vi "Initialise Chmmr.vi"(8 "error in (no error)":errorcluster, 11 "Renderer":u32) -> (0 "error out":errorcluster, 2 "Deployables":refnum<class "Zap Sat.lvclass">[](array[class]), 3 "Ship out":refnum<class "Chmmr.lvclass">)   [LabVIEW 2021, in "Chmmr.lvclass"]
uses:
  Chmmr.lvclass
  Deployables/Zap Sat/Zap Sat.lvclass
  Re-use Libraries/Vector 2D/Vector 2D.lvclass
  Ship/Config.ctl
  Ship/Ship.lvclass
  Element/Player Type.ctl
  Element/Element.lvclass
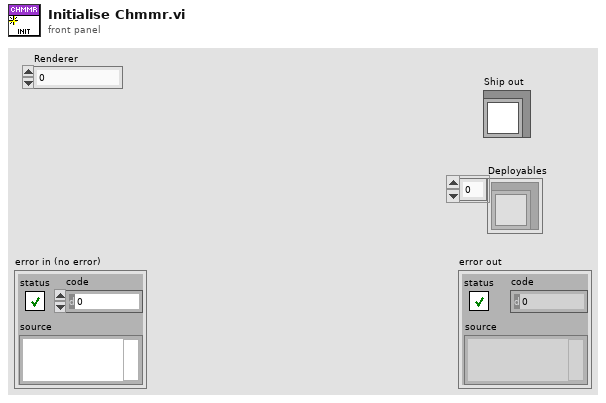
[diagram p1: front panel]
types:
  T1 = typedef "Ship.lvclass/Config.ctl" = cluster{"Race":string, "Ship Name":string, "Max Crew":i32, "Max Energy":i32, "Energy Regeneration":i32, "Weapon Energy Cost":i32, "Special Energy Cost":i32, "Energy Wait":i32, "Max Thrust":i32, "Thrust Increment":i32, "Turn Wait":i32, "Thrust Wait":i32, "Weapon Wait":i32, "Special Wait":i32, "Ship Mass":i32, "Captain Name":string}
  T2 = typedef "Constants.ctl" = cluster{"Colours":cluster{"OK":u32, "Warning":u32, "Error":u32, "Red":u32, "Green":u32, "Blue":u32, "Yellow":u32, "Health":u32, "Energy":u32}, "System":cluster{"Target Frames Second":dbl, "Windows Size":refnum<class "Vector 2D.lvclass">, "World Size":refnum<class "Vector 2D.lvclass">, "Battle Area Size":refnum<class "Vector 2D.lvclass">, "Sidebar Width":sgl, "SC2 Frame Rate [Seconds/Frame]":sgl, "Sidebar Player 2 Y Offset":sgl}, "Game":cluster{"Maximum Asteroids":i32, "Max Energy":i32, "Max Crew":i32, "Maximum Stars":i32}}
  T3 = typedef "Element.lvclass/Player Type.ctl" = enum16{"Neutral", "Player 1", "Player 2"}
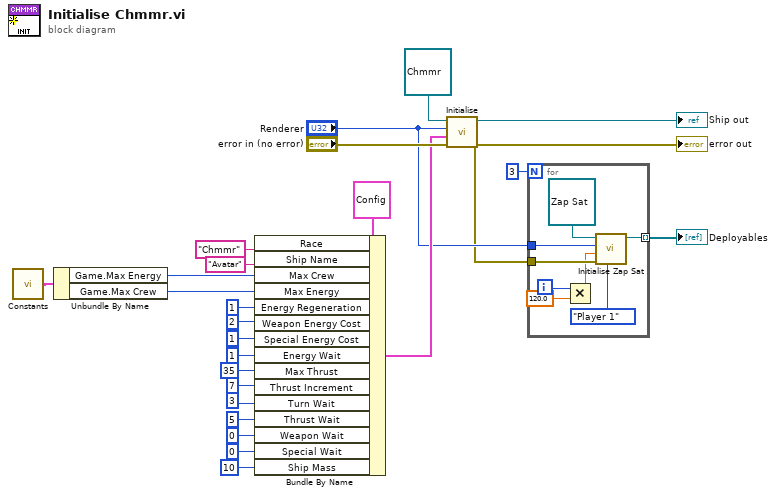
[diagram p0: block diagram]
diagram:
  n1 = call "Constants.vi"() -> ("Constants"=w24:T2)
  n2 = Unbundle By Name(w24) -> ("Game.Max Energy"=w18:i32, "Game.Max Crew"=w17:i32)
  n3 = Bundle By Name(cluster=T1 {"Race"="", "Ship Name"="", "Max Crew"=0, "Max Energy"=0, "Energy Regeneration"=0, "Weapon Energy Cost"=0, "Special Energy Cost"=0, "Energy Wait"=0, "Max Thrust"=0, "Thrust Increment"=0, "Turn Wait"=0, "Thrust Wait"=0, "Weapon Wait"=0, "Special Wait"=0, "Ship Mass"=0, "Captain Name"=""} ("Common"), "Race"="Chmmr" ("name or relative path"), "Ship Name"="Avatar", "Max Crew"=w18, "Max Energy"=w17, "Energy Regeneration"=1 ("Turn Wait"), "Weapon Energy Cost"=2 ("Turn Wait"), "Special Energy Cost"=1 ("Energy Regeneration"), "Energy Wait"=1 ("Weapon Energy Cost"), "Max Thrust"=35 ("Weapon Energy Cost"), "Thrust Increment"=7 ("Special Energy Cost"), "Turn Wait"=3 ("Energy Wait"), "Thrust Wait"=5 ("Max Thrust"), "Weapon Wait"=0 ("Thrust Increment"), "Special Wait"=0, "Ship Mass"=10) -> (w20:T1)
  n4 = call-dynamic "Initialise.vi"("error in (no error)"="error in (no error)", "Common"=w20, "Renderer"="Renderer", "Ship in"=refnum<class "Chmmr.lvclass"> refnum ("Ship")) -> ("error out"=w3:errorcluster, "Ship out"=→"Ship out":refnum<class "Chmmr.lvclass">)  [unwired: 6 in]
  "error out" <- w3
  n5 = for {
    N: 3 -> [_]
    tunnel: "Renderer" -> [w32]
    tunnel: w3 -> [w31]
    tunnel: [w30] -> w1 mode=indexing
    i -> [w29]
    n6 = Multiply(x=w29, y=sgl 120.0) -> (x*y=w27:sgl)
    n7 = call "Initialise Zap Sat.vi"("Player Type"=Player_Type."Player 1", "error in (no error)"=w31, "Angle"=w27, "Renderer"=w32, "Deployable in"=refnum<class "Zap Sat.lvclass"> refnum ("Zap Sat.lvclass")) -> ("Deployable out"=w30:refnum<class "Zap Sat.lvclass">)  [unwired: 5 in, 1 out]
  }
  "Deployables" <- w1
